vi "gfitsio-insert-col.vi"(4 "tunits":string, 6 "tform":string, 7 "ttype":string, 8 "error in (no error)":errorcluster, 10 "insertion point (0:1st column)":i32, 11 "gfits refnum":T1) -> (0 "error out":errorcluster, 3 "dup gfits refnum":T1)   [LabVIEW 2019, in "gfitsio.lvlib"]
doc: "Insert a column in an ASCII or binary table. When inserting, <B>insertion point</B> specifies the column number that the new column should occupy in the table. Any existing columns from this position and higher are shifted over to allow room for the new column(s). The index number on all the following keywords will be incremented or decremented if necessary to reflect the new position of the column(s) in the table: TBCOLn, TFORMn, TTYPEn, TUNITn, TNULLn, TSCALn, TZEROn, TDISPn, TDIMn, TLMINn, TLMAXn, TDMINn, TDMAXn, TCTYPn, TCRPXn, TCRVLn, TCDLTn, TCROTn, and TCUNIn.\n\nThe FITS Standard recommends that only letters, digits, and the underscore character be used in column names (the ttype parameter) with no embedded spaces. Trailing blank characters are not significant. It is recommended that all the column names in a given table be unique within the first 8 characters, and strongly recommended that the names be unique within the first 16 characters."
uses:
  gfitsio.lvlib
  gfitsio-refnum.ctl
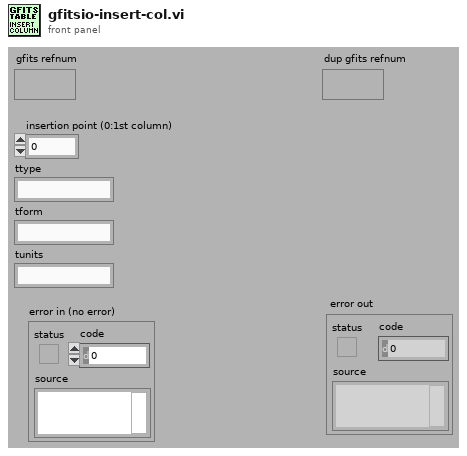
[diagram p1: front panel]
types:
  T1 = typedef "gfitsio.lvlib/gfitsio-refnum.ctl" = refnum<k1>
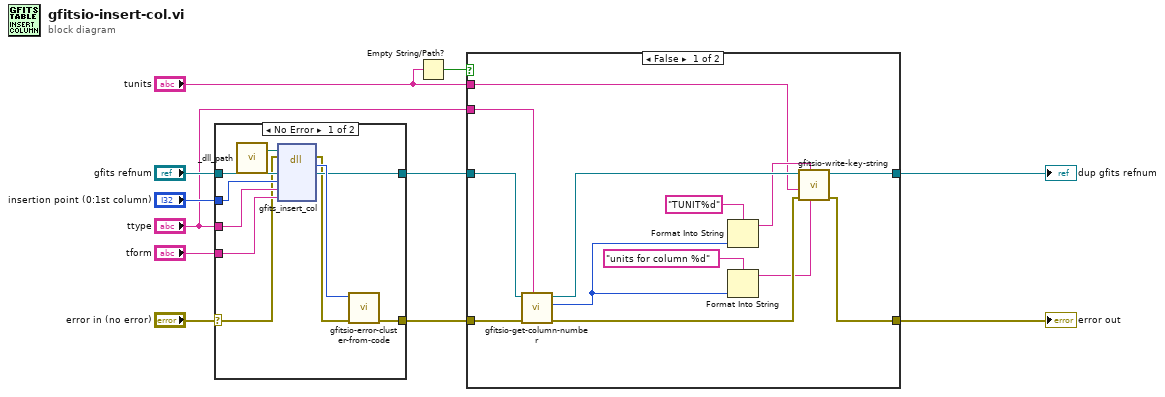
[diagram p0: block diagram]
diagram:
  n1 = case shown="No Error" "error in (no error)" {
    selector: "error in (no error)" -> [w13 w23]
    tunnel: [w21 w23] -> w4
    tunnel: "ttype" -> [w19 _]
    tunnel: "gfits refnum" -> [w17 w22]
    tunnel: [w18 w22] -> w5
    tunnel: "tform" -> [w16 _]
    tunnel: "insertion point (0:1st column)" -> [w15 _]
    frame No Error {
      n2 = call "_dll_path.vi"() -> ("Path"=w14:path)  [unwired: 1 in]
      n3 = dll-call lib="?" fn="gfits_insert_col"(path in=w14, error in=w13, "refnum"=w17, "colnum"=w15, "ttype"=w19, "tform"=w16) -> (error out=w12:errorcluster, "return type"=w20:i32, "refnum"=w18:T1)  [unwired: 4 in, 1 out]
      n4 = call "gfitsio-error-cluster-from-code.vi"("error in (no error)"=w12, "error code"=w20) -> ("error out"=w21:errorcluster)  [unwired: 9 out]
    }
    frame Error {
    }
  }
  n5 = Empty String/Path?(string/path="tunits") -> (empty?=w1:bool)
  n6 = case shown="False" w1 {
    tunnel: [w36 w37] -> w7
    tunnel: [w35 w38] -> w6
    tunnel: w5 -> [w32 w38]
    tunnel: w4 -> [w31 w37]
    tunnel: "ttype" -> [w30 _]
    tunnel: "tunits" -> [w28 _]
    frame False {
      n7 = call "gfitsio-get-column-number.vi"("column"=w30, "error in (no error)"=w31, "gfits refnum"=w32) -> ("error out"=w34:errorcluster, "colnum"=w25:i32, "dup gfits refnum"=w33:T1)  [unwired: 6 in]
      n8 = Format Into String(format string="TUNIT%d" ("value"), w25) -> (resulting string=w29:string)  [unwired: 2 in, 1 out]
      n9 = Format Into String(format string="units for column %d" ("value"), w25) -> (resulting string=w27:string)  [unwired: 2 in, 1 out]
      n10 = call "gfitsio-write-key-string.vi"("comment"=w27, "keyname"=w29, "error in (no error)"=w34, "value"=w28, "gfits refnum"=w33) -> ("error out"=w36:errorcluster, "dup gfits refnum"=w35:T1)  [unwired: 5 in]
    }
    frame True {
    }
  }
  "error out" <- w7
  "dup gfits refnum" <- w6
